vi "Image Example.vi"() -> ()   [LabVIEW 2020]
uses:
  g_ar_toolkit.common/Image Size (Integer).ctl
  g_ar_toolkit.image/CreateEmptyImageARGB.vi
  g_ar_toolkit.image/ResizeARGB.vi
  g_ar_toolkit.image/ShowWindowARGB.vi
  g_ar_toolkit.image/CopyArrayToImageARGB.vi
  g_ar_toolkit.image/CopyPixmapToImageFlattenMaskARGB.vi
  g_ar_toolkit.image/CreateEmptyImageGreyscale.vi
  g_ar_toolkit.image/DrawImageToPictureGreyscale.vi
  g_ar_toolkit.image/DrawImageWithMaskToPictureARGB.vi
  g_ar_toolkit.image/CreateEmptyImageARGB.vi/3321fa97-f432-4e1e-8db9-a0df79aed21b.vi
  g_ar_toolkit.image/ARGBColourToU32.vi
  g_ar_toolkit.image/ResizeARGB.vi/c2d955e4-7b08-44cd-801f-dcd0ae61a3f9.vi
  g_ar_toolkit.image/ShowWindowARGB.vi/df490a54-c425-41e5-8765-b6fcf549c24a.vi
  g_ar_toolkit.image/CopyArrayToImageARGB.vi/26c70cee-9332-41f4-9755-08948a885cbe.vi
  g_ar_toolkit.image/DrawImageToPictureARGB.vi/8cd07b1b-062e-4fe4-9e87-2eb3dc89fe0e.vi
  g_ar_toolkit.image/CopyPixmapToImageFlattenMaskARGB.vi/80b1166a-8c06-443b-b271-eb6a715622f7.vi
  g_ar_toolkit.image/CreateEmptyImageGreyscale.vi/6598b9e0-8a08-46f5-91fd-ca1b87217137.vi
  g_ar_toolkit.image/ARGBExtractChannel.vi
  g_ar_toolkit.image/DrawImageToPictureGreyscale.vi/9ae995ca-ccda-485c-89ac-02736fde3e8e.vi
  g_ar_toolkit.image/MaskFromColour.vi/5701baee-35e2-4306-9a77-a9fdbb5b3a7f.vi
  g_ar_toolkit.image/DrawImageWithMaskToPictureARGB.vi/8cd07b1b-062e-4fe4-9e87-2eb3dc89fe0e.vi
  g_ar_toolkit.image/FixPixmap.vi
  g_ar_toolkit.image/Default8bitColourMap.vi
  g_ar_toolkit.common/Module Path.vi
  <vilib>/Utility/error.llb/Error Cluster From Error Code.vi
  g_ar_toolkit.image/g_ar_toolkit.image.lvlib
  g_ar_toolkit.common/g_ar_toolkit.common.lvlib
panel:
  out "Image with Blue Pixels Masked":picture
  out "Copied From Pixmap and Converted To Greyscale":picture
  out "Original":picture
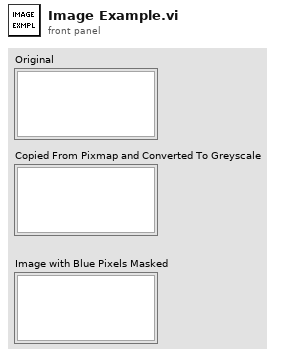
[diagram p1: front panel]
types:
  T1 = typedef "g_ar_toolkit.common.lvlib/Image Size (Integer).ctl" = cluster{"Width":u16, "Height":u16}
  T2 = typedef "imagedata.ctl" = cluster{"image type":i32, "image depth":i32, "image":u8[], "mask":u8[], "colors":u32[], "Rectangle":cluster{"left":i16, "top":i16, "right":i16, "bottom":i16}}
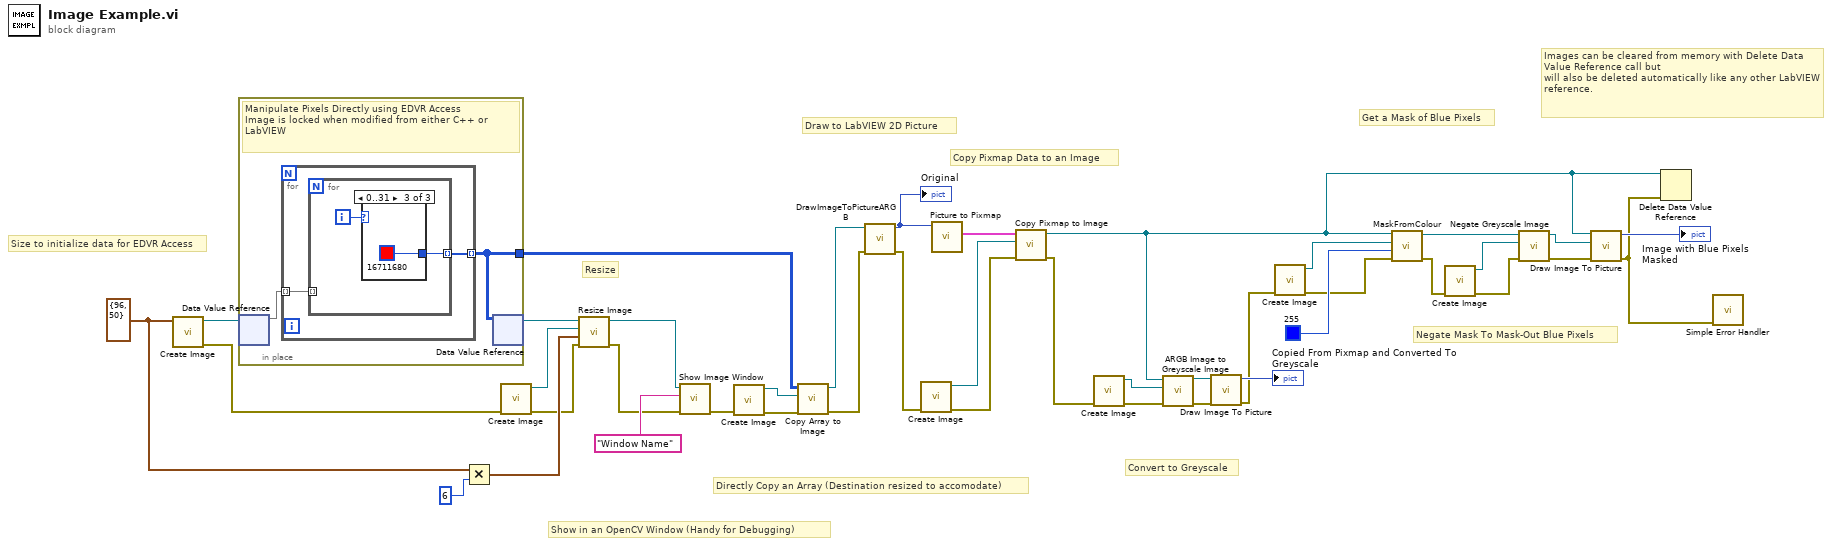
[diagram p0: block diagram]
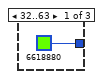
[diagram p2: hidden frame]
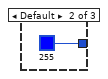
[diagram p3: hidden frame]
diagram:
  w1 = T1 {"Width"=96, "Height"=50} ("Preallocated Image Size (Default: 0,0)")
  # "Directly Copy an Array (Destination resized to accomodate)"
  # "Images can be cleared from memory with Delete Data Value Reference call but\nwill also be deleted automatically like any other LabVIEW reference."
  # "Convert to Greyscale"
  # "Copy Pixmap Data to an Image"
  # "Draw to LabVIEW 2D Picture"
  # "Show in an OpenCV Window (Handy for Debugging)"
  # "Resize"
  # "Size to initialize data for EDVR Access"
  # "Negate Mask To Mask-Out Blue Pixels"
  # "Get a Mask of Blue Pixels"
  n1 = call-poly "Create Image.vi"("Preallocated Image Size (Default: 0,0)"=w1) -> ("error out"=w36:errorcluster, "New ARGB Image"=w41:refnum<data-value>)  [unwired: 9 in]
  n2 = in-place {
    in-place-border: [w42] -> w6
    # "Manipulate Pixels Directly using EDVR Access\nImage is locked when modified from either C++ or LabVIEW"
    n3 = in-place-dvr #1(w41) -> (w43:u32[][])  [unwired: 1 out]
    n4 = for {
      tunnel: w43 -> [w45] mode=indexing
      tunnel: [w44] -> w42 mode=indexing
      n5 = for {
        tunnel: w45 -> [_] mode=indexing
        tunnel: [w46] -> w44 mode=indexing
        i -> [w47]
        n6 = case shown="0..31" w47 {
          tunnel: [u32 6618880 u32 255 u32 16711680] -> w46
          frame 32..63 {
          }
          frame Default {
          }
          frame 0..31 {
          }
        }
      }
    }
    n7 = in-place-dvr #1(w42) -> (w33:refnum<data-value>)  [unwired: 1 out]
  }
  n8 = Multiply(x=w1, y=u16 6) -> (x*y=w39:T1)
  n9 = call-poly "Create Image.vi"("error in (no error)"=w36) -> ("error out"=w35:errorcluster, "New ARGB Image"=w38:refnum<data-value>)  [unwired: 9 in]
  n10 = call-poly "Resize Image.vi"("error in (no error)"=w35, "New Image Size"=w39, "ARGB Destination Image"=w38, "ARGB Source Image"=w33) -> ("error out"=w34:errorcluster, "ARGB  Destination Image (duplicate)"=w32:refnum<data-value>)  [unwired: 6 in]
  n11 = call-poly "Show Image Window.vi"("error in (no error)"=w34, "Window Name"="Window Name", "ARGB Image"=w32) -> ("error out"=w9:errorcluster)  [unwired: 7 in, 1 out]
  n12 = call-poly "Create Image.vi"("error in (no error)"=w9) -> ("error out"=w8:errorcluster, "New ARGB Image"=w7:refnum<data-value>)  [unwired: 9 in]
  n13 = call-poly "Copy Array to Image.vi"("error in (no error)"=w8, "ARGB Image Destination"=w7, "Source"=w6) -> ("error out"=w4:errorcluster, "ARGB Image Destination (Duplicate)"=w5:refnum<data-value>)  [unwired: 7 in]
  n14 = call "DrawImageToPictureARGB.vi"("error in (no error)"=w4, "ARGB Image Source"=w5) -> ("error out"=w28:errorcluster, "Picture"=w31:picture)  [unwired: 8 in]
  "Original" <- w31
  n15 = call-poly "Create Image.vi"("error in (no error)"=w28) -> ("error out"=w27:errorcluster, "New ARGB Image"=w29:refnum<data-value>)  [unwired: 9 in]
  n16 = call <vilib>:"Picture to Pixmap.vi"("picture"=w31) -> ("image data"=w30:T2)  [unwired: 9 in, 1 out]
  n17 = call-poly "Copy Pixmap to Image.vi"("error in (no error)"=w27, "ARGB Image Destination"=w29, "Pixmap Image Data"=w30) -> ("error out"=w25:errorcluster, "ARGB Image Destination (duplicate)"=w3:refnum<data-value>)  [unwired: 7 in]
  n18 = call-poly "Create Image.vi"("error in (no error)"=w25) -> ("error out"=w26:errorcluster, "New Greyscale Image"=w24:refnum<data-value>)  [unwired: 9 in]
  n19 = call "ARGB Image to Greyscale Image.vi"("error in (no error)"=w26, "Greyscale Image Destination"=w24, "ARGB Image Source"=w3) -> ("error out"=w23:errorcluster, "Greyscale Image Destination (Duplicate)"=w22:refnum<data-value>)  [unwired: 7 in]
  n20 = call-poly "Draw Image To Picture.vi"("error in (no error)"=w23, "Greyscale Image Source"=w22) -> ("error out"=w20:errorcluster, "Picture"=→"Copied From Pixmap and Converted To Greyscale":picture)  [unwired: 8 in]
  n21 = call-poly "Create Image.vi"("error in (no error)"=w20) -> ("error out"=w2:errorcluster, "New Greyscale Image"=w19:refnum<data-value>)  [unwired: 9 in]
  n22 = call "MaskFromColour.vi"("error in (no error)"=w2, "Value"=u32 255, "Mask Destination"=w19, "ARGB Image Source"=w3) -> ("error out"=w15:errorcluster, "Mask Destination (duplicate)"=w14:refnum<data-value>)  [unwired: 6 in]
  n23 = call-poly "Create Image.vi"("error in (no error)"=w15) -> ("error out"=w12:errorcluster, "New Greyscale Image"=w11:refnum<data-value>)  [unwired: 9 in]
  n24 = call "Negate Greyscale Image.vi"("error in (no error)"=w12, "Greyscale Image-Destination"=w11, "Greyscale Image-Source"=w14) -> ("error out"=w16:errorcluster, "Greyscale Image-Destination (duplicate)"=w13:refnum<data-value>)  [unwired: 7 in]
  n25 = call-poly "Draw Image To Picture.vi"("error in (no error)"=w16, "Greyscale Mask"=w13, "ARGB Image Source"=w3) -> ("error out"=w10:errorcluster, "Picture"=→"Image with Blue Pixels Masked":picture)  [unwired: 7 in]
  n26 = Delete Data Value Reference(data value reference=w3, error in=w10) -> ()  [unwired: 2 out]
  n27 = call <vilib>:"Simple Error Handler.vi"("error in (no error)"=w10) -> ()  [unwired: 4 in, 5 out]
